vi "PWM_Test_v1.vi"(9 "HMP4040 VISA":refnum<visa-resource-name>="HMP4040_FTS2", 10 "ControlBoard VISA":refnum<visa-resource-name>="ControlBoard", 11 "Board Selector":T1) -> (3 "Result (bool)":bool)   [LabVIEW 2019]
uses:
  Ctls/Powersupply_Auto_Enum_v1.ctl
  <vilib>/DAQmx/read.llb/DAQmx Read (Analog 1D Wfm NChan NSamp).vi
  Ctls/Controlboard_Select.ctl
panel:
  in  "error in (no error)":errorcluster
  out "ControlBoard OUT":refnum<visa-resource-name>
  in  "Message IN":string=" "
  out "Message OUT":string
  out "Active Leg":i32
  out "Waveforms":T2
  out "Analysis Leg":i32
  out "error out":errorcluster
  out "Result (color)":u32(colorbox)
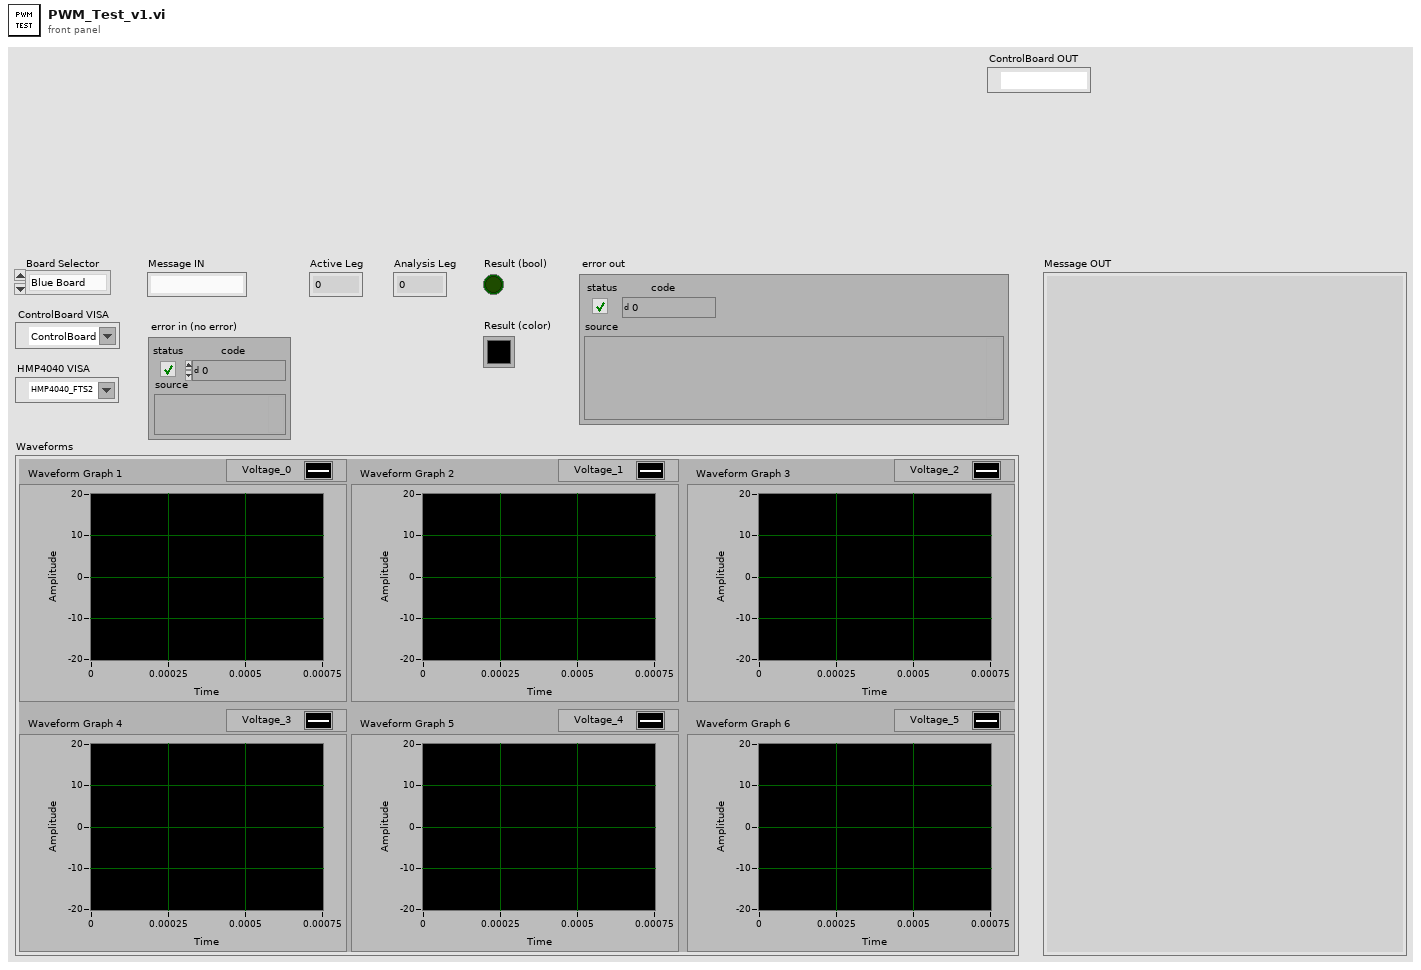
[diagram p1: front panel]
types:
  T1 = typedef "Controlboard_Select.ctl" = enum16{"Blue Board", "Green Board"}
  T2 = cluster{"Waveform Graph 1":waveform(dbl), "Waveform Graph 2":waveform(dbl), "Waveform Graph 3":waveform(dbl), "Waveform Graph 4":waveform(dbl), "Waveform Graph 5":waveform(dbl), "Waveform Graph 6":waveform(dbl)}
  T3 = typedef "Powersupply_Auto_Enum_v1.ctl" = enum16{"Off", "Control Power", "HMP2020 Control + DC32V", "HMP2020 Control + DC8V", "HMP4040 Control + DC32V", "HMP4040 Control +DC8V"}
  T4 = cluster{"data[0]":waveform(dbl), "data[1]":waveform(dbl), "data[2]":waveform(dbl), "data[3]":waveform(dbl), "data[4]":waveform(dbl), "data[5]":waveform(dbl)}
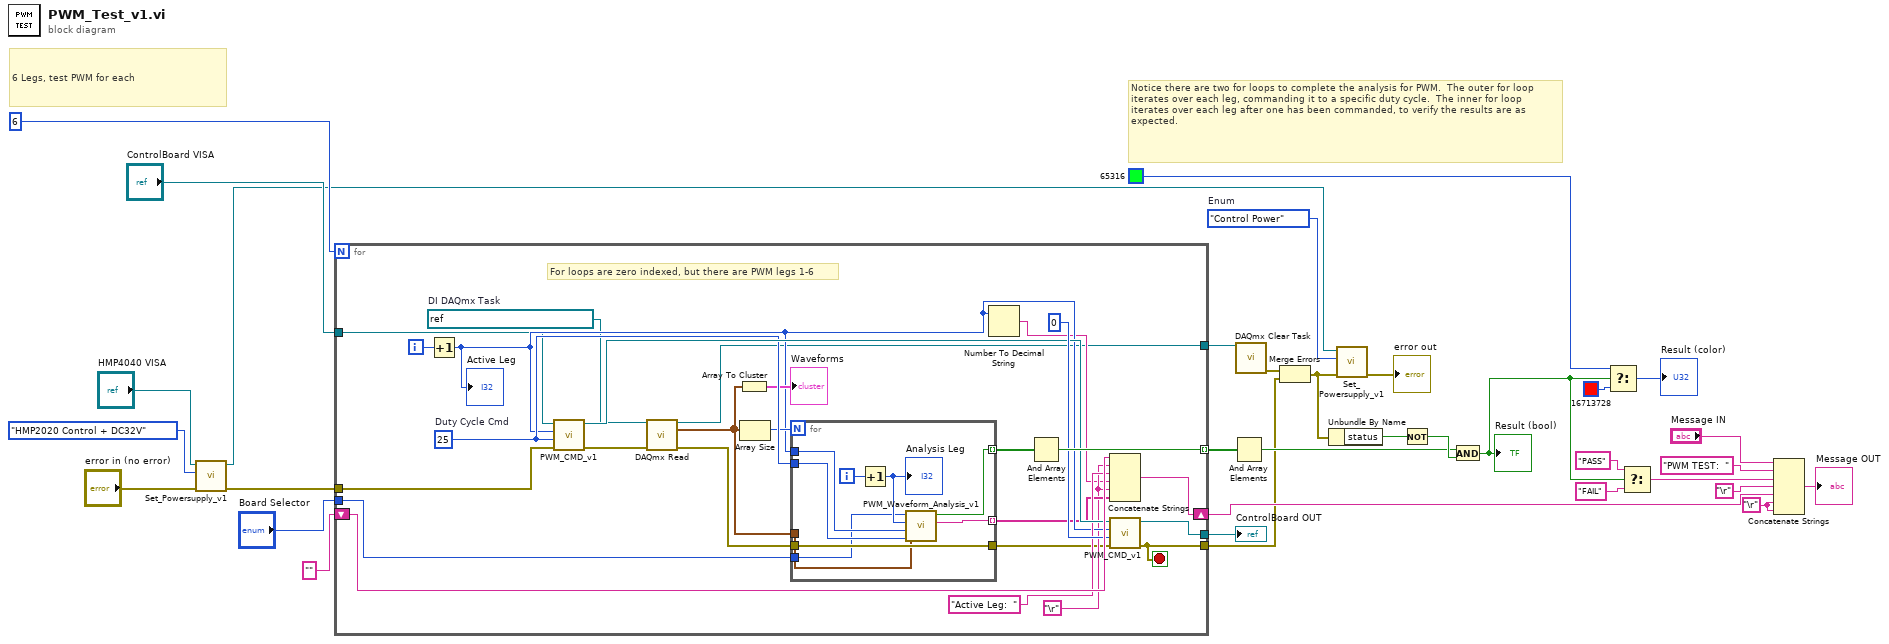
[diagram p0: block diagram]
diagram:
  w8 = Powersupply_Auto_Enum_v1."Control Power"  # Enum
  w22 = "\r"
  # "Notice there are two for loops to complete the analysis for PWM.  The outer for loop iterates over each leg, commanding it to a specific duty cycle.  The inner for loop iterates over each leg after one has been commanded, to verify the results are as expected."
  # "6 Legs, test PWM for each"
  n1 = call "Set_Powersupply_v1.vi"("error in (no error)"="error in (no error)", "Enum"=Powersupply_Auto_Enum_v1."HMP2020 Control + DC32V", "HMP VISA"="HMP4040 VISA") -> ("error out"=w6:errorcluster, "HMP VISA Out"=w7:refnum<visa-resource-name>)  [unwired: 7 in]
  n2 = for {
    N: 6 -> [_]
    tunnel: "ControlBoard VISA" -> [w39]
    tunnel: [w59] -> w33 mode=indexing
    shift-right: [w57] -> w20
    shift-left: "" -> [w56]
    tunnel: w6 -> [w58]
    tunnel: [w51] -> w5
    tunnel: [w46] -> w18
    tunnel: [w36] -> w2
    tunnel: "Board Selector" -> [w35]
    i -> [w52]
    stop <- w51 stop-if-true
    w34 = refnum<k21> "BTS_PWMInput_Hydra_CB"  # DI DAQmx Task
    w41 = "\r"
    w53 = 25  # Duty Cycle Cmd
    # "For loops are zero indexed, but there are PWM legs 1-6"
    n3 = Increment(x=w52) -> (x+1=w43:i32)
    "Active Leg" <- w43
    n4 = call "PWM_CMD_v1.vi"("error in (no error)"=w58, "Duty Cycle"=w53, "Leg"=w43, "VISA Refnum in"=w39) -> ("error out"=w45:errorcluster, "VISA Refnum out"=w54:refnum<visa-resource-name>)  [unwired: 6 in]
    n5 = call-poly <vilib>:"DAQmx Read.vi"("task/channels in"=w34, "error in"=w45) -> ("task out"=w36:refnum<k21>, "data"=w47:waveform(dbl)[], "error out"=w38:errorcluster)  [unwired: 11 in]
    n6 = Array To Cluster(array=w47) -> (cluster=→"Waveforms":T4)
    n7 = Array Size(array=w47) -> (size(s)=w48:i32)
    n8 = for {
      N: w48 -> [_]
      tunnel: w53 -> [w68]
      tunnel: w47 -> [w63]
      tunnel: w43 -> [w67]
      tunnel: [w60] -> w49 mode=indexing
      tunnel: [w62] -> w42 mode=indexing
      tunnel: w38 -> [w64]
      tunnel: [w64] -> w37
      tunnel: w35 -> [w61]
      i -> [w66]
      n9 = Increment(x=w66) -> (x+1=w65:i32)
      "Analysis Leg" <- w65
      n10 = call "PWM_Waveform_Analysis_v1.vi"("Waveform"=w63, "Duty Cycle"=w68, "Active Leg"=w67, "Analysis Leg"=w65, 11:w61) -> ("Message"=w62:string, "Result (Boolean)"=w60:bool)  [unwired: 5 in]
    }
    n11 = Number To Decimal String(number=w43) -> (decimal integer string=w40:string)  [unwired: 1 in]
    n12 = And Array Elements(Boolean array=w49) -> (logical AND=w59:bool)
    n13 = Concatenate Strings(w56, w41, "Active Leg:  ", w40, w41, w42) -> (w57:string)
    n14 = call "PWM_CMD_v1.vi"("error in (no error)"=w37, "Duty Cycle"=0, "Leg"=w43, "VISA Refnum in"=w54) -> ("error out"=w51:errorcluster, "VISA Refnum out"=w46:refnum<visa-resource-name>)  [unwired: 6 in]
  }
  "ControlBoard OUT" <- w18
  n15 = And Array Elements(Boolean array=w33) -> (logical AND=w23:bool)
  n16 = call <vilib>:"DAQmx Clear Task.vi"("task in"=w2) -> ("error out"=w1:errorcluster)  [unwired: 14 in]
  n17 = Merge Errors(w1, w5) -> (w12:errorcluster)
  n18 = Unbundle By Name(w12) -> ("status"=w26:bool)
  n19 = call "Set_Powersupply_v1.vi"("error in (no error)"=w12, "Enum"=w8, "HMP VISA"=w7) -> ("error out"=→"error out":errorcluster)  [unwired: 7 in, 1 out]
  n20 = Not(x=w26) -> (.not. x?=w25:bool)
  n21 = And(x=w23, y=w25) -> (x .and. y?=w24:bool)
  "Result (bool)" <- w24
  n22 = Select(t=u32 65316 ("Result (color)"), s=w24, f=u32 16713728 ("Result (color)")) -> (s? t:f=→"Result (color)":u32)
  n23 = Select(t="PASS", s=w24, f="FAIL") -> (s? t:f=w14:string)
  n24 = Concatenate Strings("Message IN", "PWM TEST:  ", w14, "\r", w20, w22, w22) -> (→"Message OUT":string)
